vi "Constants.vi"() -> (4 "VI path":path, 6 "Exe script name":string="TestforEXETemplate.vi", 8 "Test folder name":string="TestforEXETemplate.vi", 10 "Script folder name":string="TestforEXETemplate.vi")   [LabVIEW 2016]
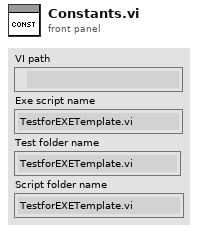
[diagram p1: front panel]
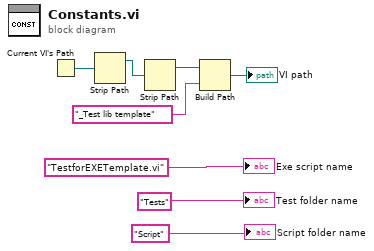
[diagram p0: block diagram]
diagram:
  n1 = Current VI's Path() -> (path=w6:path)
  n2 = Strip Path(path=w6) -> (stripped path=w1:path)  [unwired: 1 out]
  n3 = Strip Path(path=w1) -> (stripped path=w2:path)  [unwired: 1 out]
  n4 = Build Path(base path=w2, name or relative path="_Test lib template") -> (appended path=→"VI path":path)
  "Exe script name" <- "TestforEXETemplate.vi" ("name or relative path")
  "Test folder name" <- "Tests" ("name or relative path")
  "Script folder name" <- "Script" ("name or relative path")
